vi "setUp.vi"(8 "error in (no error)":errorcluster, 11 "reference in":refnum<class "SLSC Switch Messaging Tests.lvclass">) -> (0 "error out":errorcluster, 3 "reference out":refnum<class "SLSC Switch Messaging Tests.lvclass">)   [LabVIEW 2017, in "SLSC Switch Messaging Tests.lvclass"]
doc: "setUp runs prior to the test method during test execution. Use this method to initialize any object data required by your tests."
uses:
  SLSC Switch Messaging Tests.lvclass
  C:/Program Files (x86)/National Instruments/LabVIEW 2017/vi.lib/addons/_JKI Toolkits/VI Tester/TestCase.llb/TestCase.lvclass
  Includes/CDMessaging.lvlibp/Producer/Abstract Producer/Abstract Producer.lvclass
  Includes/CDMessaging.lvlibp/Parameters/Abstract Init Parameters/Abstract Init Parameters.lvclass
  SLSC Switch Init Parameters/SLSC Switch Init Parameters.lvclass
  C:/Dev/GitHub/niveristand-slsc-switch-message-library/Includes/CDMessaging.lvlibp/Parameters/Abstract Init Parameters/Abstract Init Parameters.lvclass
  C:/Dev/GitHub/niveristand-slsc-switch-message-library/Includes/CDMessaging.lvlibp/Switch/Abstract Switch Init Parameters/Abstract Switch Init Parameters.lvclass
  Includes/CDMessaging.lvlibp/Message Queue/Message Queue/Message Queue.lvclass
  C:/Dev/GitHub/niveristand-slsc-switch-message-library/Includes/CDMessaging.lvlibp/Message Queue/Abstract Message Queue/Abstract Message Queue.lvclass
  Support/Mock SLSC Switch Consumer.lvclass
  C:/Dev/GitHub/niveristand-slsc-switch-message-library/Includes/CDMessaging.lvlibp/Switch/Abstract Switch Consumer/Abstract Switch Consumer.lvclass
  SLSC Switch Messaging Tests.lvclass/SLSC Switch Messaging Tests.ctl
  <userlib>/_OpenG.lib/file/file.llb/Append Path to Root if Relative - Scalar__ogtk.vi
  <vilib>/addons/_JKI Toolkits/VI Tester/TestCase.llb/TestCase.lvclass
  Includes/CDMessaging.lvlibp/Consumer/Abstract Consumer/Abstract Consumer.lvclass
  niveristand-custom-device-testing-tools/VeriStandTestUtilities/VeriStandTestUtilities.lvlib
  C:/Dev/GitHub/niveristand-slsc-switch-message-library/Includes/CDMessaging.lvlibp/Consumer/Abstract Consumer/Abstract Consumer.lvclass
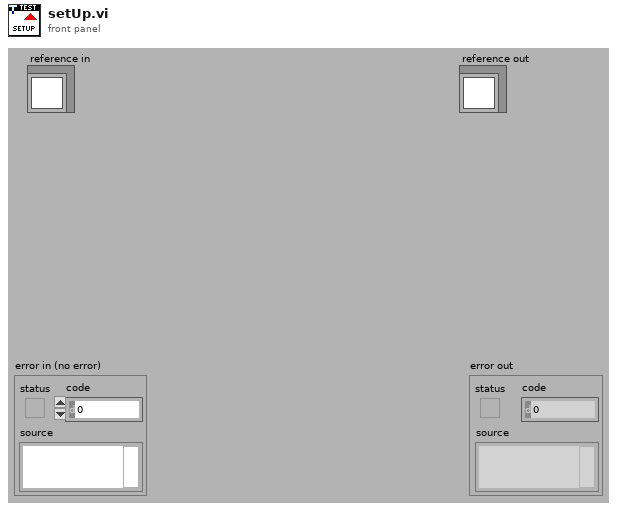
[diagram p1: front panel]
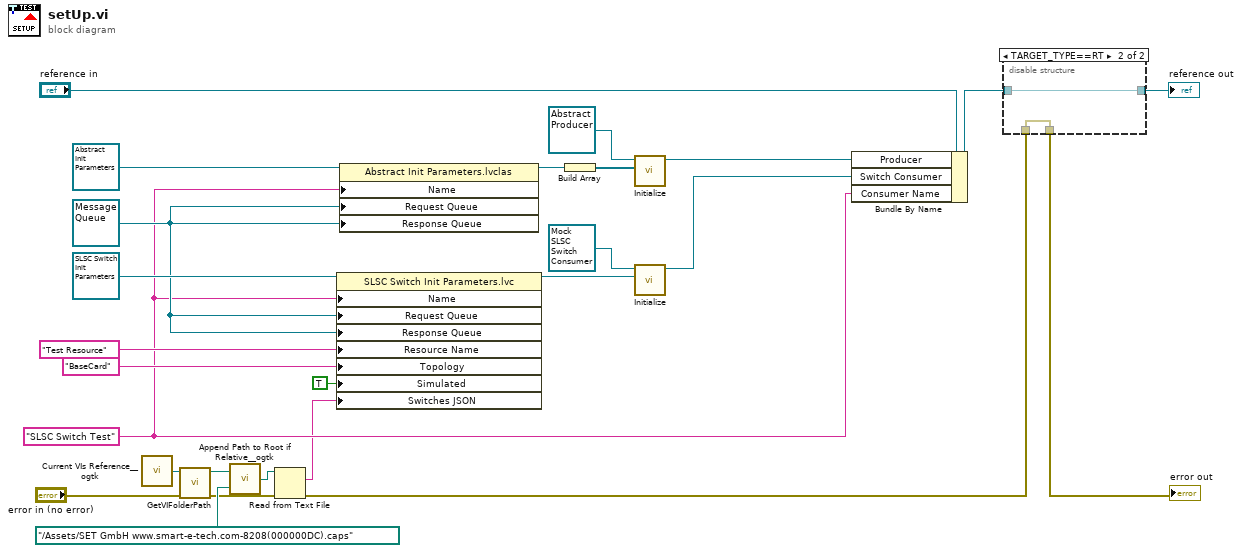
[diagram p0: block diagram]
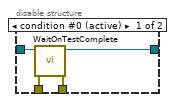
[diagram p2: hidden frame]
diagram:
  w10 = "SLSC Switch Test"
  w20 = refnum<class "Message Queue.lvclass"> refnum ("CDMessaging.lvlibp:Message Queue.lvclass")
  n1 = call <userlib>:"Current VIs Reference__ogtk.vi"() -> ("Current VI's reference"=w9:refnum<vi>)  [unwired: 5 in]
  n2 = call "GetVIFolderPath.vi"("error in (no error)"="error in (no error)", "VI Reference in"=w9) -> ("error out"=w4:errorcluster, "VI Folder Path out"=w8:path)  [unwired: 8 in]
  n3 = call-poly <userlib>:"Append Path to Root if Relative__ogtk.vi"("Absolute or Relative Path"=path "../Assets/SET GmbH www.smart-e-tech.com-8208(000000DC).caps" ("Capabilities File"), "Root Path"=w8) -> ("Absolute or Appended Path"=w2:path)
  n4 = Read from Text File(file (use dialog)=w2, error in=w4) -> (text=w1:string, error out=w3:errorcluster)  [unwired: 2 in, 2 out]
  n5 = property class="SLSC Switch Init Parameters.lvc"(reference=refnum<class "SLSC Switch Init Parameters.lvclass"> refnum ("SLSC Switch Messaging.lvlib:SLSC Switch Init Parameters.lvclass"), "Name"=w10, "Request Queue"=w20, "Response Queue"=w20, "Resource Name"="Test Resource", "Topology"="BaseCard", "Simulated"=TRUE, "Switches JSON"=w1) -> (reference out=w13:refnum<class "SLSC Switch Init Parameters.lvclass">)  [unwired: 1 in, 1 out]
  n6 = property class="Abstract Init Parameters.lvclas"(reference=refnum<class "Abstract Init Parameters.lvclass"> refnum ("CDMessaging.lvlibp:Abstract Init Parameters.lvclass"), "Name"=w10, "Request Queue"=w20, "Response Queue"=w20) -> (reference out=w16:refnum<class "Abstract Init Parameters.lvclass">)  [unwired: 1 in, 1 out]
  n7 = Build Array(w16) -> (w15:refnum<class "Abstract Init Parameters.lvclass">[])
  n8 = call "Initialize.vi"("Parameters in"=w15, "Abstract Producer in"=refnum<class "Abstract Producer.lvclass"> refnum ("CDMessaging.lvlibp:Abstract Producer.lvclass")) -> ("Abstract Producer out"=w12:refnum<class "Abstract Producer.lvclass">)  [unwired: 8 in, 1 out]
  n9 = call "Initialize.vi"("Parameters in"=w13, "Abstract Consumer in"=refnum<class "Mock SLSC Switch Consumer.lvclass"> refnum ("Mock SLSC Switch Consumer.lvclass")) -> ("Abstract Consumer out"=w11:refnum<class "Mock SLSC Switch Consumer.lvclass">)  [unwired: 8 in, 1 out]
  n10 = Bundle By Name(cluster="reference in", "Producer"=w12, "Switch Consumer"=w11, "Consumer Name"=w10) -> (w23:refnum<class "SLSC Switch Messaging Tests.lvclass">)
  n11 = disable-structure shown="TARGET_TYPE==RT" {
    disable-tunnel: w3 -> [w30 w31]
    disable-tunnel: [w29 w31] -> w26
    disable-tunnel: [w28 w32] -> w24
    disable-tunnel: w23 -> [w27 w32]
    frame condition #0 (active) {
      n12 = call <vilib>:"WaitOnTestComplete.vi"("error in (no error)"=w30, "TestCase in"=w27) -> ("error out"=w29:errorcluster, "TestCase out"=w28:refnum<class "SLSC Switch Messaging Tests.lvclass">)  [unwired: 8 in]
    }
    frame condition #1 {
    }
  }
  "error out" <- w26
  "reference out" <- w24
